vi "Konfig changes.vi"(8 "Fehler (Eingang, kein Fehler)":errorcluster, 10 "TestKonfig alt":T2 {"TestKonfig Interferent"."Gasflasche MFC3" items=["----"=10000, "IAG NH3 3000"=0, "IAG NH3 200"=1, "IAG NH3 2000"=2, "IAG MG"=3, "IAG O2"=4]; "TestKonfig Interferent"."Gasflasche MFC2" items=["----"=10000, "IAG NH3 3000"=0, "IAG NH3 200"=1, "IAG NH3 2000"=2, "IAG MG"=3, "IAG O2"=4]; "TestKonfig Interferent"."Eingangs Konzentration MFC1" min=0.0; "TestKonfig Interferent"."Ausgangs Konzentration MFC1" min=0.0; "TestKonfig Interferent"."MFC2" items=["MFC 2", "MFC 3", "MFC 4", "MFC 5"]; "TestKonfig Interferent"."MFC3" items=["MFC 2", "MFC 3", "MFC 4", "MFC 5"]; "TestKonfig Interferent"."Ausgangs Konzentration MFC3" min=0.0; "TestKonfig Interferent"."Eingangs Konzentration MFC3" min=0.0; "TestKonfig Interferent"."Ausgangs Konzentration MFC2" min=0.0; "TestKonfig Interferent"."Eingangs Konzentration MFC2" min=0.0; "TestKonfig H2O"."HovaCAL Temperature" format="%.2f"; "TestKonfig H2O"."HovaCAL Flow Input Cluster"."HovaCAL Flow Input Cluster" format="%.2f"; "TestKonfig H2O"."Eingangs Konzentration:" min=0.0; "TestKonfig H2O"."zusätzliche Zeitdauer Erster Punkt" min=30 step=1 format="%#_5g"; "TestKonfig H2O"."Zeitdauer Stufen" format="%#_5g"; "TestKonfig H2O"."Max Fehler" format="%#_5g"; "TestKonfig H2O"."Anzahl Stufen" format="%#_5g"; "TestKonfig H2O"."Modus" items=["Messen", "CG zu Entnahmestelle"]}, 11 "TestKonfig (Eingang)":T2 {"TestKonfig Interferent"."Gasflasche MFC3" items=["----"=10000, "IAG NH3 3000"=0, "IAG NH3 200"=1, "IAG NH3 2000"=2, "IAG MG"=3, "IAG O2"=4]; "TestKonfig Interferent"."Gasflasche MFC2" items=["----"=10000, "IAG NH3 3000"=0, "IAG NH3 200"=1, "IAG NH3 2000"=2, "IAG MG"=3, "IAG O2"=4]; "TestKonfig Interferent"."Eingangs Konzentration MFC1" min=0.0; "TestKonfig Interferent"."Ausgangs Konzentration MFC1" min=0.0; "TestKonfig Interferent"."MFC2" items=["MFC 2", "MFC 3", "MFC 4", "MFC 5"]; "TestKonfig Interferent"."MFC3" items=["MFC 2", "MFC 3", "MFC 4", "MFC 5"]; "TestKonfig Interferent"."Ausgangs Konzentration MFC3" min=0.0; "TestKonfig Interferent"."Eingangs Konzentration MFC3" min=0.0; "TestKonfig Interferent"."Ausgangs Konzentration MFC2" min=0.0; "TestKonfig Interferent"."Eingangs Konzentration MFC2" min=0.0; "TestKonfig H2O"."HovaCAL Temperature" format="%.2f"; "TestKonfig H2O"."HovaCAL Flow Input Cluster"."HovaCAL Flow Input Cluster" format="%.2f"; "TestKonfig H2O"."Eingangs Konzentration:" min=0.0; "TestKonfig H2O"."zusätzliche Zeitdauer Erster Punkt" min=30 step=1 format="%#_5g"; "TestKonfig H2O"."Zeitdauer Stufen" format="%#_5g"; "TestKonfig H2O"."Max Fehler" format="%#_5g"; "TestKonfig H2O"."Anzahl Stufen" format="%#_5g"; "TestKonfig H2O"."Modus" items=["Messen", "CG zu Entnahmestelle"]}) -> (0 "Fehler (Ausgang)":errorcluster, 1 "Changes":T12, 2 "TestKonfig alt out":T2 {"TestKonfig Interferent"."Gasflasche MFC3" items=["----"=10000, "IAG NH3 3000"=0, "IAG NH3 200"=1, "IAG NH3 2000"=2, "IAG MG"=3, "IAG O2"=4]; "TestKonfig Interferent"."Gasflasche MFC2" items=["----"=10000, "IAG NH3 3000"=0, "IAG NH3 200"=1, "IAG NH3 2000"=2, "IAG MG"=3, "IAG O2"=4]; "TestKonfig Interferent"."Eingangs Konzentration MFC1" min=0.0; "TestKonfig Interferent"."Ausgangs Konzentration MFC1" min=0.0; "TestKonfig Interferent"."MFC2" items=["MFC 2", "MFC 3", "MFC 4", "MFC 5"]; "TestKonfig Interferent"."MFC3" items=["MFC 2", "MFC 3", "MFC 4", "MFC 5"]; "TestKonfig Interferent"."Ausgangs Konzentration MFC3" min=0.0; "TestKonfig Interferent"."Eingangs Konzentration MFC3" min=0.0; "TestKonfig Interferent"."Ausgangs Konzentration MFC2" min=0.0; "TestKonfig Interferent"."Eingangs Konzentration MFC2" min=0.0; "TestKonfig H2O"."HovaCAL Temperature" format="%.2f"; "TestKonfig H2O"."HovaCAL Flow Input Cluster"."HovaCAL Flow Input Cluster" format="%.2f"; "TestKonfig H2O"."Eingangs Konzentration:" min=0.0; "TestKonfig H2O"."zusätzliche Zeitdauer Erster Punkt" min=30 step=1 format="%#_5g"; "TestKonfig H2O"."Zeitdauer Stufen" format="%#_5g"; "TestKonfig H2O"."Max Fehler" format="%#_5g"; "TestKonfig H2O"."Anzahl Stufen" format="%#_5g"; "TestKonfig H2O"."Modus" items=["Messen", "CG zu Entnahmestelle"]}, 3 "TestKonfig (Ausgang)":T2 {"TestKonfig Interferent"."Gasflasche MFC3" items=["----"=10000, "IAG NH3 3000"=0, "IAG NH3 200"=1, "IAG NH3 2000"=2, "IAG MG"=3, "IAG O2"=4]; "TestKonfig Interferent"."Gasflasche MFC2" items=["----"=10000, "IAG NH3 3000"=0, "IAG NH3 200"=1, "IAG NH3 2000"=2, "IAG MG"=3, "IAG O2"=4]; "TestKonfig Interferent"."Eingangs Konzentration MFC1" min=0.0; "TestKonfig Interferent"."Ausgangs Konzentration MFC1" min=0.0; "TestKonfig Interferent"."MFC2" items=["MFC 2", "MFC 3", "MFC 4", "MFC 5"]; "TestKonfig Interferent"."MFC3" items=["MFC 2", "MFC 3", "MFC 4", "MFC 5"]; "TestKonfig Interferent"."Ausgangs Konzentration MFC3" min=0.0; "TestKonfig Interferent"."Eingangs Konzentration MFC3" min=0.0; "TestKonfig Interferent"."Ausgangs Konzentration MFC2" min=0.0; "TestKonfig Interferent"."Eingangs Konzentration MFC2" min=0.0; "TestKonfig H2O"."HovaCAL Temperature" format="%.2f"; "TestKonfig H2O"."HovaCAL Flow Input Cluster"."HovaCAL Flow Input Cluster" format="%.2f"; "TestKonfig H2O"."Eingangs Konzentration:" min=0.0; "TestKonfig H2O"."zusätzliche Zeitdauer Erster Punkt" min=30 step=1 format="%#_5g"; "TestKonfig H2O"."Zeitdauer Stufen" format="%#_5g"; "TestKonfig H2O"."Max Fehler" format="%#_5g"; "TestKonfig H2O"."Anzahl Stufen" format="%#_5g"; "TestKonfig H2O"."Modus" items=["Messen", "CG zu Entnahmestelle"]}, 4 "Einheiten Changes-Cluster":T1, 5 "changed":bool)   [LabVIEW 2020, in "EPA 1065.lvlib" / "HovaCAL Interference verificaton.lvlib"]
uses:
  HovaCAL Interference verificaton.lvlib
  TestKonfig.ctl
  TestKonfig H2O.ctl
  Modus.ctl
  Linearisierung V2/SpanEinstellungen/Einheit.ctl
  Linearisierung V2/Gasteiler/Stufen Tabelle 10 Stufen.ctl
  Linearisierung V2/Gasteiler/HovaCAL_Interface/Controls/Flow Einstellung.ctl
  Linearisierung V2/Gasteiler/HovaCAL_Interface/Controls/Temp Sollwerte Anzeige.ctl
  TestKonfig Interferents.ctl
  MFCAuswahl.ctl
  Seiten/System Einstellungen V2/Gasflasche Auswahl.ctl
  Konfig changes.ctl
  Seiten/System Einstellungen V2/System Einstellungen V2.lvlib
  Linearisierung V2/SpanEinstellungen/SpanEinstellungen.lvlib
  Linearisierung V2/Gasteiler/HovaCAL_Interface/Controls/Controls.lvlib
  Linearisierung V2/Gasteiler/Gasteiler.lvlib
panel:
  # "sec"
  # "%"
  # "sec"
  # "sec"
  # "%"
  # "sec"
  # "sec"
  # "%"
  # "sec"
  # "sec"
  # "%"
  # "sec"
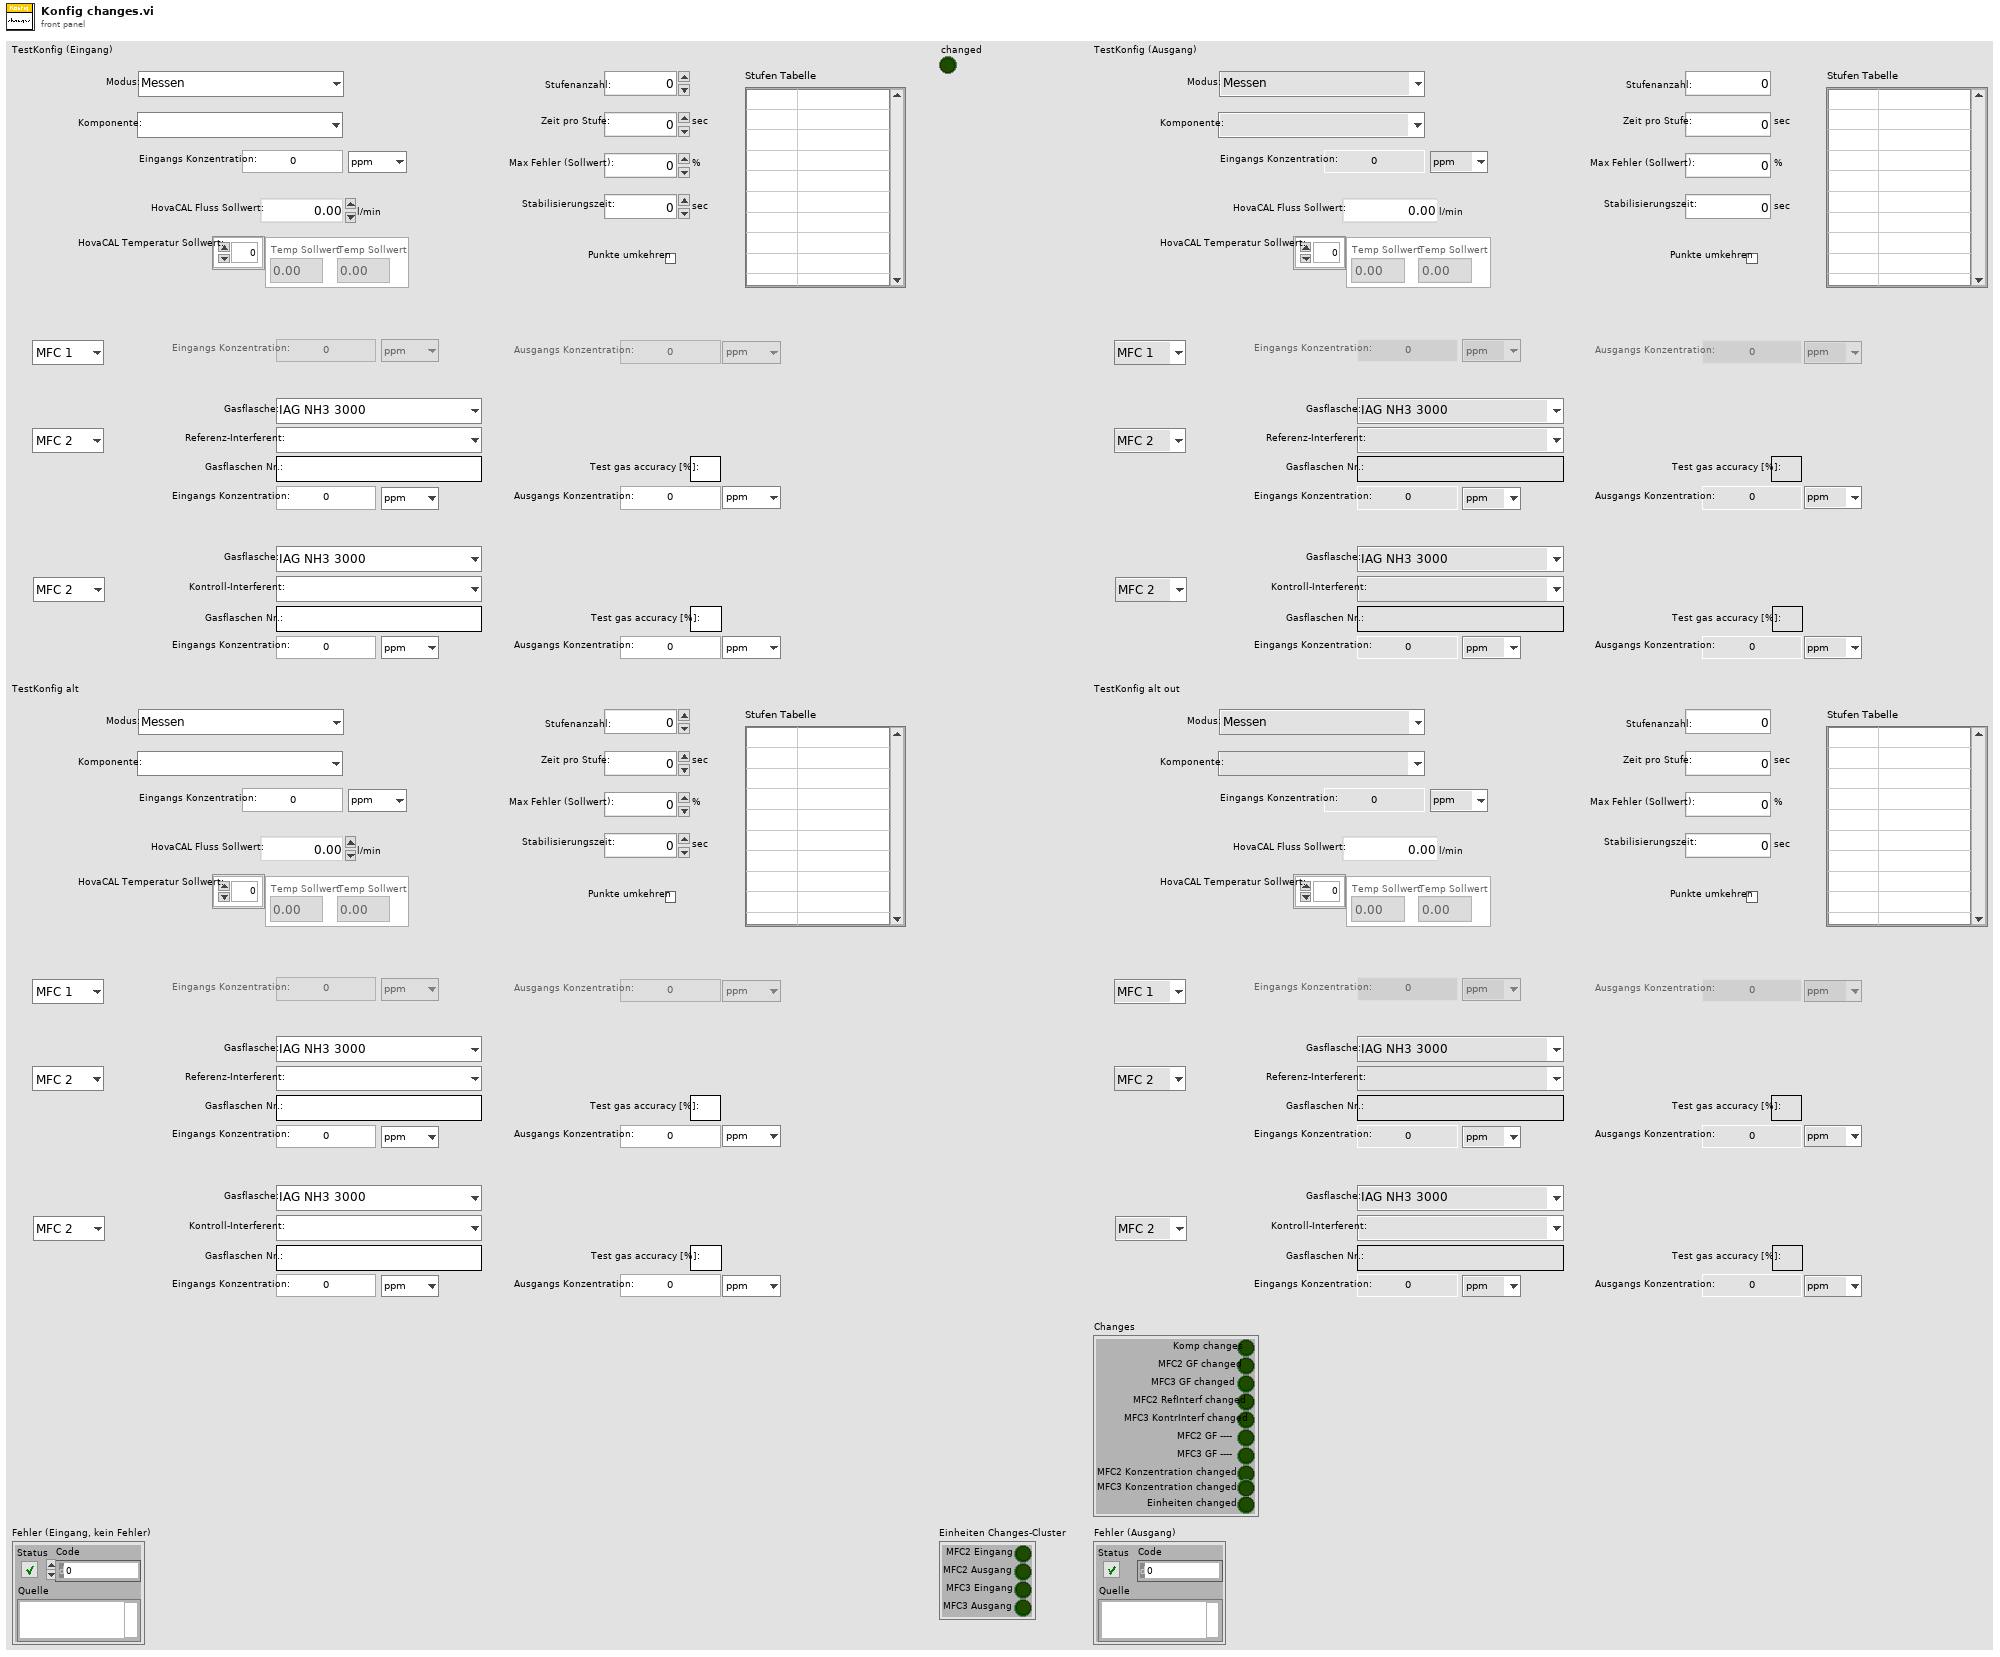
[diagram p1: front panel]
types:
  T1 = cluster{"MFC2 Eingang":bool, "MFC2 Ausgang":bool, "MFC3 Eingang":bool, "MFC3 Ausgang":bool}
  T2 = typedef "EPA 1065.lvlib/HovaCAL Interference verificaton.lvlib/TestKonfig.ctl" = cluster{"TestKonfig H2O":T3, "TestKonfig Interferent":T9}
  T3 = typedef "EPA 1065.lvlib/HovaCAL Interference verificaton.lvlib/TestKonfig H2O.ctl" = cluster{"Modus":T4, "Komponente:":u16, "Eingangs Konzentration:":dbl, "Einheit":T5, "Anzahl Stufen":sgl, "Zeitdauer Stufen":sgl, "Max Fehler":sgl, "zusätzliche Zeitdauer Erster Punkt":sgl, "Punkte umkehren":bool, "Stufen Tabelle":T6, "HovaCAL Flow Input Cluster":T7, "HovaCAL Temperature":T8}
  T4 = typedef "EPA 1065.lvlib/HovaCAL Interference verificaton.lvlib/Modus.ctl" = u16
  T5 = typedef "Linearisierung v2.lvlib/SpanEinstellungen.lvlib/Einheit.ctl" = enum16{"ppm", "%"}
  T6 = typedef "Linearisierung v2.lvlib/Gasteiler.lvlib/Stufen Tabelle 10 Stufen.ctl" = string[][]
  T7 = typedef "Linearisierung v2.lvlib/Gasteiler.lvlib/HovaCAL_Interface.lvlib/Controls.lvlib/Flow Einstellung.ctl" = cluster{"HovaCAL Flow Input Cluster":dbl}
  T8 = typedef "Linearisierung v2.lvlib/Gasteiler.lvlib/HovaCAL_Interface.lvlib/Controls.lvlib/Temp Sollwerte Anzeige.ctl" = dbl[]
  T9 = typedef "EPA 1065.lvlib/HovaCAL Interference verificaton.lvlib/TestKonfig Interferents.ctl" = cluster{"MFC1":enum16{"MFC 1"}, "Eingangs Konzentration MFC1":dbl, "Einheit MFC1 Eingang":T5, "Ausgangs Konzentration MFC1":dbl, "Einheit MFC1 Ausgang":T5, "MFC2":T10, "Referenz-Interferent:":u16, "Gasflaschen Nr MFC2":string, "Accuracy MFC2":string, "Eingangs Konzentration MFC2":dbl, "Einheit MFC2 Eingang":T5, "Ausgangs Konzentration MFC2":dbl, "Einheit MFC2 Ausgang":T5, "MFC3":T10, "Kontroll-Interferent:":u16, "Gasflaschen Nr MFC3":string, "Accuracy MFC3":string, "Eingangs Konzentration MFC3":dbl, "Einheit MFC3 Eingang":T5, "Ausgangs Konzentration MFC3":dbl, "Einheit MFC3 Ausgang":T5, "Gasflasche MFC2":T11, "Gasflasche MFC3":T11}
  T10 = typedef "EPA 1065.lvlib/HovaCAL Interference verificaton.lvlib/MFCAuswahl.ctl" = u16
  T11 = typedef "System Einstellungen V2.lvlib/Gasflasche Auswahl.ctl" = u16
  T12 = typedef "EPA 1065.lvlib/HovaCAL Interference verificaton.lvlib/Konfig changes.ctl" = cluster{"Komp changes":bool, "MFC2 GF changed":bool, "MFC3 GF changed":bool, "MFC2 RefInterf changed":bool, "MFC3 KontrInterf changed":bool, "MFC2 GF ----":bool, "MFC3 GF ----":bool, "MFC2 Konzentration changed":bool, "MFC3 Konzentration changed":bool, "Einheiten changed":bool}
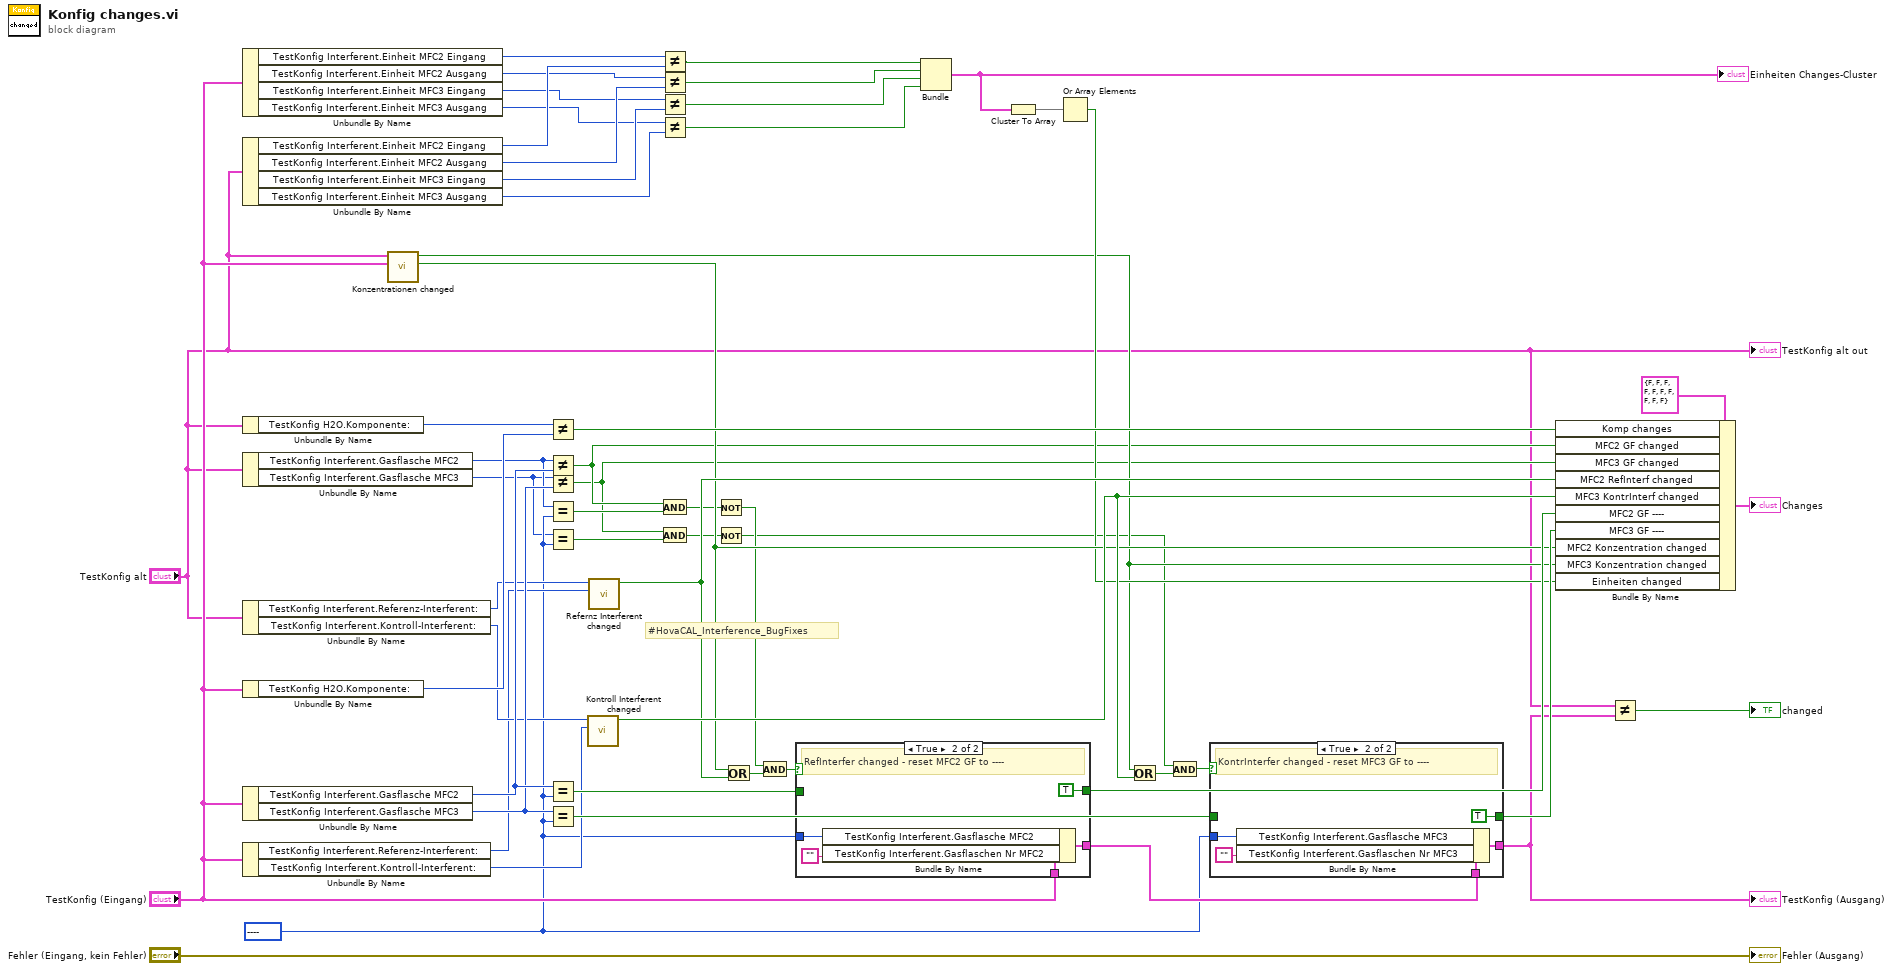
[diagram p0: block diagram]
diagram:
  w10 = T11 10000 items=["----"=10000, "IAG NH3 3000"=0, "IAG NH3 200"=1, "IAG NH3 2000"=2, "IAG MG"=3, "IAG O2"=4] ("Gasflasche MFC2")
  # "#HovaCAL_Interference_BugFixes"
  n1 = Unbundle By Name("TestKonfig (Eingang)") -> ("TestKonfig Interferent.Einheit MFC2 Eingang"=w35:T5, "TestKonfig Interferent.Einheit MFC2 Ausgang"=w33:T5, "TestKonfig Interferent.Einheit MFC3 Eingang"=w31:T5, "TestKonfig Interferent.Einheit MFC3 Ausgang"=w29:T5)
  n2 = Unbundle By Name("TestKonfig alt") -> ("TestKonfig Interferent.Einheit MFC2 Eingang"=w34:T5, "TestKonfig Interferent.Einheit MFC2 Ausgang"=w32:T5, "TestKonfig Interferent.Einheit MFC3 Eingang"=w30:T5, "TestKonfig Interferent.Einheit MFC3 Ausgang"=w28:T5)
  n3 = Unbundle By Name("TestKonfig alt") -> ("TestKonfig H2O.Komponente:"=w54:u16)
  n4 = Unbundle By Name("TestKonfig alt") -> ("TestKonfig Interferent.Gasflasche MFC2"=w15:T11, "TestKonfig Interferent.Gasflasche MFC3"=w9:T11)
  n5 = Unbundle By Name("TestKonfig alt") -> ("TestKonfig Interferent.Referenz-Interferent:"=w39:u16, "TestKonfig Interferent.Kontroll-Interferent:"=w40:u16)
  n6 = Unbundle By Name("TestKonfig (Eingang)") -> ("TestKonfig H2O.Komponente:"=w55:u16)
  n7 = Unbundle By Name("TestKonfig (Eingang)") -> ("TestKonfig Interferent.Gasflasche MFC2"=w51:T11, "TestKonfig Interferent.Gasflasche MFC3"=w50:T11)
  n8 = Unbundle By Name("TestKonfig (Eingang)") -> ("TestKonfig Interferent.Referenz-Interferent:"=w38:u16, "TestKonfig Interferent.Kontroll-Interferent:"=w41:u16)
  n9 = call "Konzentrationen changed.vi"("TestKonfig (Eingang)"="TestKonfig (Eingang)", "TestKonfig alt"="TestKonfig alt") -> ("MFC2 changed"=w19:bool, "MFC3 changed"=w17:bool)  [unwired: 8 in]
  n10 = Not Equal?(x=w54, y=w55) -> (x != y?=w53:bool)
  n11 = Not Equal?(x=w15, y=w51) -> (x != y?=w16:bool)
  n12 = Not Equal?(x=w9, y=w50) -> (x != y?=w6:bool)
  n13 = Equal?(x=w15, y=w10) -> (x = y?=w11:bool)
  n14 = Equal?(x=w9, y=w10) -> (x = y?=w5:bool)
  n15 = Equal?(x=w51, y=w10) -> (x = y?=w49:bool)
  n16 = Equal?(x=w50, y=w10) -> (x = y?=w48:bool)
  n17 = call "Kontroll Interferent changed.vi"("Kontroll-Interferent:"=w41, "Kontroll-Interferent: alt"=w40) -> ("geändert"=w42:bool)  [unwired: 9 in]
  n18 = call "Refernz Interferent changed.vi"("Referenz-Interferent:"=w38, "Referenz-Interferent: alt"=w39) -> ("geändert"=w37:bool)  [unwired: 9 in]
  n19 = Not Equal?(x=w35, y=w34) -> (x != y?=w26:bool)
  n20 = Not Equal?(x=w33, y=w32) -> (x != y?=w27:bool)
  n21 = Not Equal?(x=w31, y=w30) -> (x != y?=w25:bool)
  n22 = Not Equal?(x=w29, y=w28) -> (x != y?=w24:bool)
  n23 = And(x=w16, y=w11) -> (x .and. y?=w7:bool)
  n24 = And(x=w6, y=w5) -> (x .and. y?=w8:bool)
  n25 = Not(x=w7) -> (.not. x?=w12:bool)
  n26 = Not(x=w8) -> (.not. x?=w4:bool)
  n27 = Or(x=w19, y=w37) -> (x .or. y?=w21:bool)
  n28 = And(x=w12, y=w21) -> (x .and. y?=w14:bool)
  n29 = case shown="True" w14 {
    tunnel: "TestKonfig (Eingang)" -> [w57 w62]
    tunnel: [w57 w61] -> w52
    tunnel: w10 -> [_ w60]
    tunnel: w49 -> [w56 _]
    tunnel: [w56 TRUE] -> w47
    frame False {
    }
    frame True {
      # "RefInterfer changed - reset MFC2 GF to ----"
      n30 = Bundle By Name(cluster=w62, "TestKonfig Interferent.Gasflasche MFC2"=w60, "TestKonfig Interferent.Gasflaschen Nr MFC2"="") -> (w61:T2)
    }
  }
  n31 = Bundle(w26, w27, w25, w24) -> (w23:cluster{bool, bool, bool, bool})  [unwired: 1 in]
  "Einheiten Changes-Cluster" <- w23
  n32 = Cluster To Array(cluster=w23) -> (array=w22:bool[])
  n33 = Or Array Elements(Boolean array=w22) -> (logical OR=w18:bool)
  n34 = Or(x=w17, y=w42) -> (x .or. y?=w20:bool)
  n35 = And(x=w4, y=w20) -> (x .and. y?=w13:bool)
  n36 = case shown="True" w13 {
    tunnel: w52 -> [w64 w69]
    tunnel: [w64 w68] -> w3
    tunnel: w10 -> [_ w67]
    tunnel: w48 -> [w63 _]
    tunnel: [w63 TRUE] -> w46
    frame False {
    }
    frame True {
      # "KontrInterfer changed - reset MFC3 GF to ----"
      n37 = Bundle By Name(cluster=w69, "TestKonfig Interferent.Gasflasche MFC3"=w67, "TestKonfig Interferent.Gasflaschen Nr MFC3"="") -> (w68:T2)
    }
  }
  "TestKonfig (Ausgang)" <- w3
  n38 = Bundle By Name(cluster=T12 {"Komp changes"=FALSE, "MFC2 GF changed"=FALSE, "MFC3 GF changed"=FALSE, "MFC2 RefInterf changed"=FALSE, "MFC3 KontrInterf changed"=FALSE, "MFC2 GF ----"=FALSE, "MFC3 GF ----"=FALSE, "MFC2 Konzentration changed"=FALSE, "MFC3 Konzentration changed"=FALSE, "Einheiten changed"=FALSE} ("Changes"), "Komp changes"=w53, "MFC2 GF changed"=w16, "MFC3 GF changed"=w6, "MFC2 RefInterf changed"=w37, "MFC3 KontrInterf changed"=w42, "MFC2 GF ----"=w47, "MFC3 GF ----"=w46, "MFC2 Konzentration changed"=w19, "MFC3 Konzentration changed"=w17, "Einheiten changed"=w18) -> (→"Changes":T12)
  n39 = Not Equal?(x="TestKonfig alt", y=w3) -> (x != y?=→"changed":bool)
  "TestKonfig alt out" <- "TestKonfig alt"
  "Fehler (Ausgang)" <- "Fehler (Eingang, kein Fehler)"
